vi "Test MQTT-4.7.3-1.vi"(8 "error in (no error)":errorcluster) -> (0 "error out":errorcluster)   [LabVIEW 2013]
uses:
  <vilib>/addons/_JKI Toolkits/Caraya/classes/Test/Test.lvclass
  source/Server/TopicFilter/TopicFilter.lvclass
  <vilib>/addons/_JKI Toolkits/Caraya/classes/Assert/Assert.lvclass
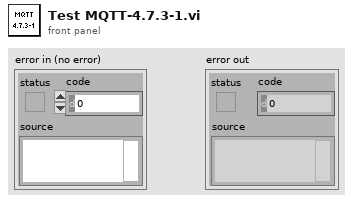
[diagram p1: front panel]
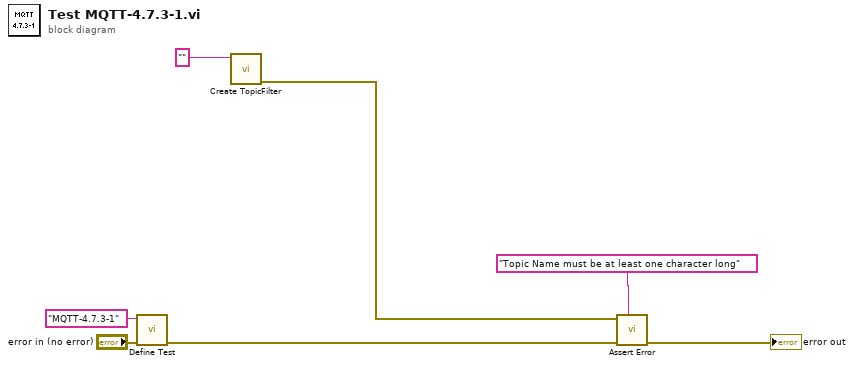
[diagram p0: block diagram]
diagram:
  n1 = call <vilib>:"Define Test.vi"("error in (no error)"="error in (no error)", "Label (VI Title)"="MQTT-4.7.3-1") -> ("error out"=w4:errorcluster)  [unwired: 9 in]
  n2 = call "Create TopicFilter.vi"("Topic Filter"="") -> ("error out"=w1:errorcluster)  [unwired: 9 in, 1 out]
  n3 = call <vilib>:"Assert Error.vi"("Label"="Topic Name must be at least one character long", "error in (no error)"=w4, "Error?"=w1) -> ("error out"=→"error out":errorcluster)  [unwired: 8 in]
